vi "CreateNewConfig.vi"(11 "error in (no error)":errorcluster) -> (0 "error out":errorcluster, 3 "Config File Path":path)   [LabVIEW 2009]
doc: "When call the DAQNavi Wizard at first, Create a blank config xml file to deliver to the wizard."
uses:
  Windows/System32/AdvLvDaq.dll
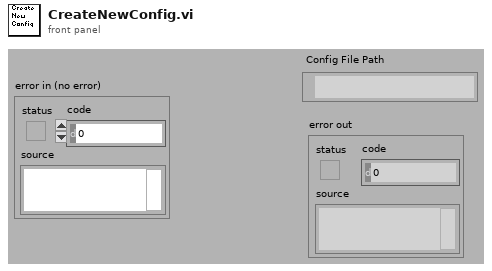
[diagram p1: front panel]
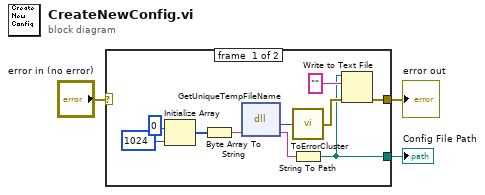
[diagram p0: block diagram]
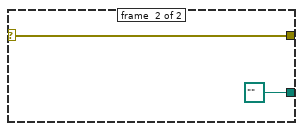
[diagram p2: hidden frame]
diagram:
  n1 = case shown="No Error" "error in (no error)" {
    selector: "error in (no error)" -> [_ w15]
    tunnel: [w13 w15] -> w2
    tunnel: [w4 path "" ("appended path")] -> w1
    frame #0 {
      n2 = Initialize Array(u8 0 ("element"), 1024 ("dimension size")) -> (w9:u8[])
      n3 = Byte Array To String(unsigned byte array=w9) -> (string=w8:string)
      n4 = dll-call lib="C:/Windows/System32/AdvLvDaq.dll" fn="GetUniqueTempFileName"("tempFileName"=w8) -> ("return type"=w6:i32, "tempFileName"=w7:string)  [unwired: 3 in, 2 out]
      n5 = call <userlib>:"ToErrorCluster.vi"("error code"=w6) -> ("error out"=w5:errorcluster)
      n6 = String To Path(string=w7) -> (path=w4:path)
      n7 = Write to Text File(file (use dialog)=w4, text="", error in=w5) -> (error out=w13:errorcluster)  [unwired: 3 out]
    }
    frame #1 {
    }
  }
  "error out" <- w2
  "Config File Path" <- w1
